vi "python_pattern_script_node.vi"(1 "Pattern Definition":T1={"Spot pitch (pixels)"=23.1, "Tilt Angle (deg)"=0.0, "Horizontal Offset (pixels)"=91.9, "Vertical Offset (pixels)"=14.1, "# Horizontal Spots"=8, "# Vertical Spots"=1, "Spot size (pixels)"=23.1, "Darken center spot"=FALSE, "Exact Phase Formula"=TRUE, "phase wrapping"=FALSE, "Set Focus (mm)"=32.0, "Add phase"=4.0, "phase_factor"=65.0, "Steering LW"=2.0, "Steering vmax"=0.0, "phase_overshoot"=TRUE, "Focal shift param"=0.0, "x0 focal shift"=0.0, "y0 focal shift"=0.0, "hv_steering"=TRUE, "fixed"=TRUE, "Pad"=0.0, "dark_all"=FALSE, "nospot"=FALSE, "Laser wavelength"=6.28e-07} {"Laser wavelength" min=0.0 max=500.0 format="%^#.3e"; "Pad" min=0.0 max=500.0 step=1.0 format="%#.0g"; "y0 focal shift" min=0.0 max=500.0 format="%#.3g"; "x0 focal shift" min=0.0 max=500.0 format="%#.3g"; "Focal shift param" min=0.0 max=500.0 format="%#.3g"; "Steering vmax" min=0.0 max=500.0 format="%#.3g"; "Steering LW" min=0.0 max=500.0 format="%#.3g"; "phase_factor" min=0.0 max=500.0 format="%#.3f"; "Add phase" min=0.0 max=500.0 format="%#.3f"; "Set Focus (mm)" min=0.0 max=500.0 format="%#.3g"; "Spot size (pixels)" min=1.0 format="%.2g"; "# Vertical Spots" min=1 step=1; "# Horizontal Spots" min=1 step=1; "Vertical Offset (pixels)" format="%.2f"; "Horizontal Offset (pixels)" format="%.2f"; "Tilt Angle (deg)" min=-90.0 max=90.0 format="%.2g"; "Spot pitch (pixels)" min=1.0 format="%.2g"}) -> (0 "Float Matrix":dbl[][](array[numeric]))   [LabVIEW 2011]
uses:
  Periodic Spot Pattern Parameters.ctl
  Periodic Spot Pattern Parameters2.ctl
panel:
  in  "center_spot (to be darkened)":u16=4
  in  "error in":errorcluster
  out "A string returned from the ScriptNode (debugging)":string="C:\\Data\\Antonio\\software\\LCOS\\LCOS"
  out "Xm":dbl[](array[numeric])=[21.72, 44.87, 68.2, 91.45, 114.72, 137.87, 160.97, 184.04]
  in  "Xm String (csv)":string="21.72,  44.87,  68.20,  91.45, 114.72, 137.87, 160.97, 184.04"
  out "Ym":dbl[](array[numeric])=[13.84, 13.78, 13.79, 13.83, 13.75, 13.79, 13.74, 13.68]
  in  "Ym String (csv)":string="13.84,  13.78,  13.79,  13.83,  13.75,  13.79,  13.74,  13.68"
  out "Intensity Graph":dbl[][](graph)
  out "error out":errorcluster
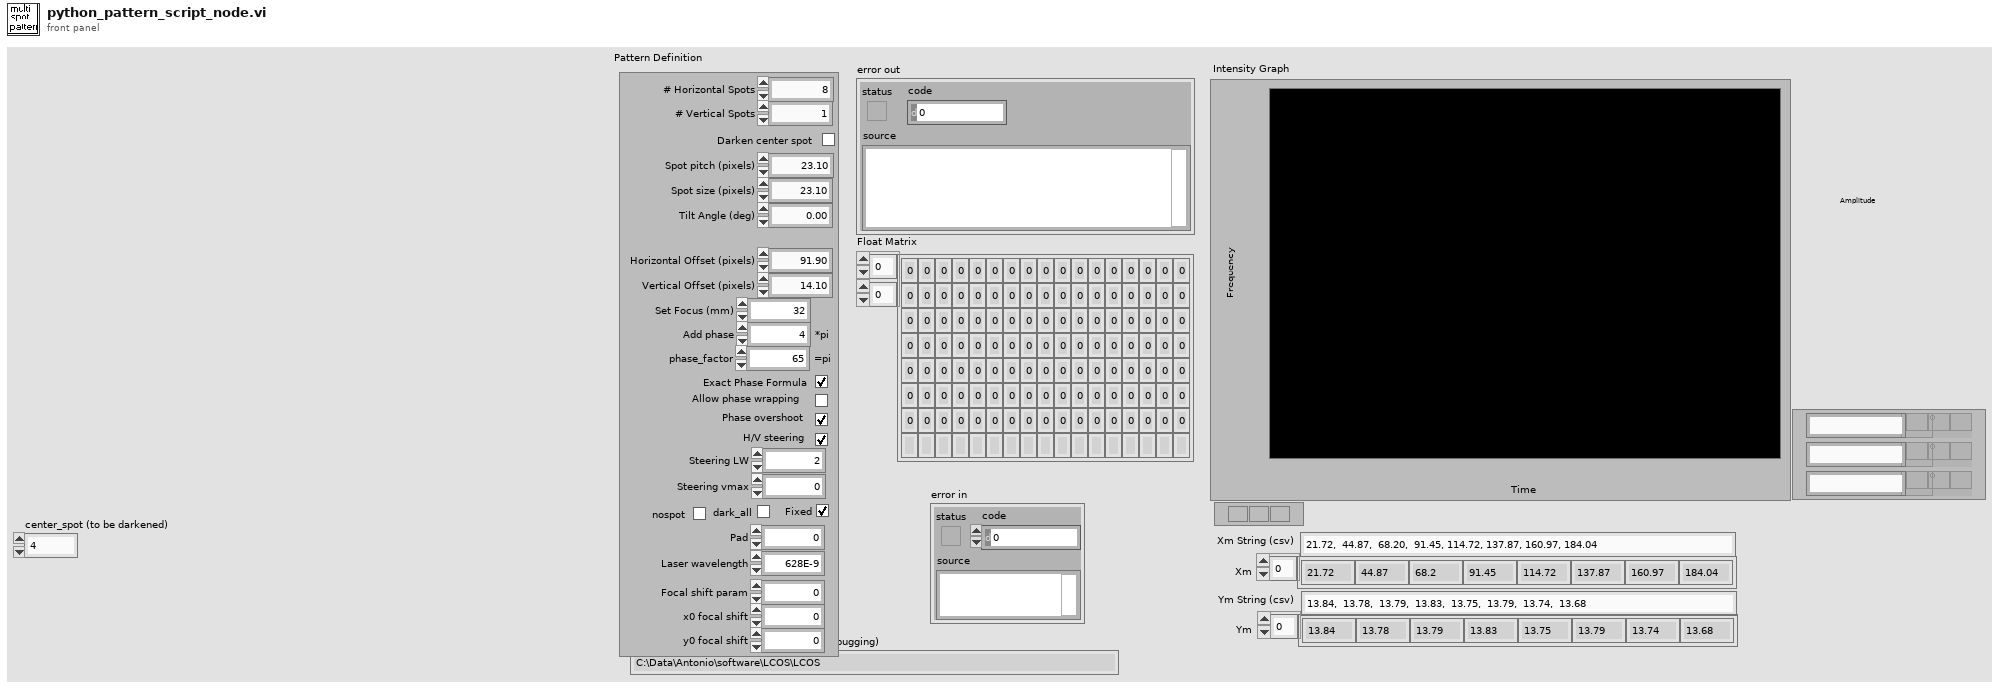
[diagram p1: front panel]
types:
  T1 = typedef "Periodic Spot Pattern Parameters.ctl" = cluster{"Spot pitch (pixels)":dbl, "Tilt Angle (deg)":dbl, "Horizontal Offset (pixels)":dbl, "Vertical Offset (pixels)":dbl, "# Horizontal Spots":u32, "# Vertical Spots":u32, "Spot size (pixels)":dbl, "Darken center spot":bool, "Exact Phase Formula":bool, "phase wrapping":bool, "Set Focus (mm)":T2, "Add phase":dbl, "phase_factor":dbl, "Steering LW":T2, "Steering vmax":T2, "phase_overshoot":bool, "Focal shift param":T2, "x0 focal shift":T2, "y0 focal shift":T2, "hv_steering":bool, "fixed":bool, "Pad":T2, "dark_all":bool, "nospot":bool, "Laser wavelength":dbl}
  T2 = typedef "Periodic Spot Pattern Parameters2.ctl" = dbl
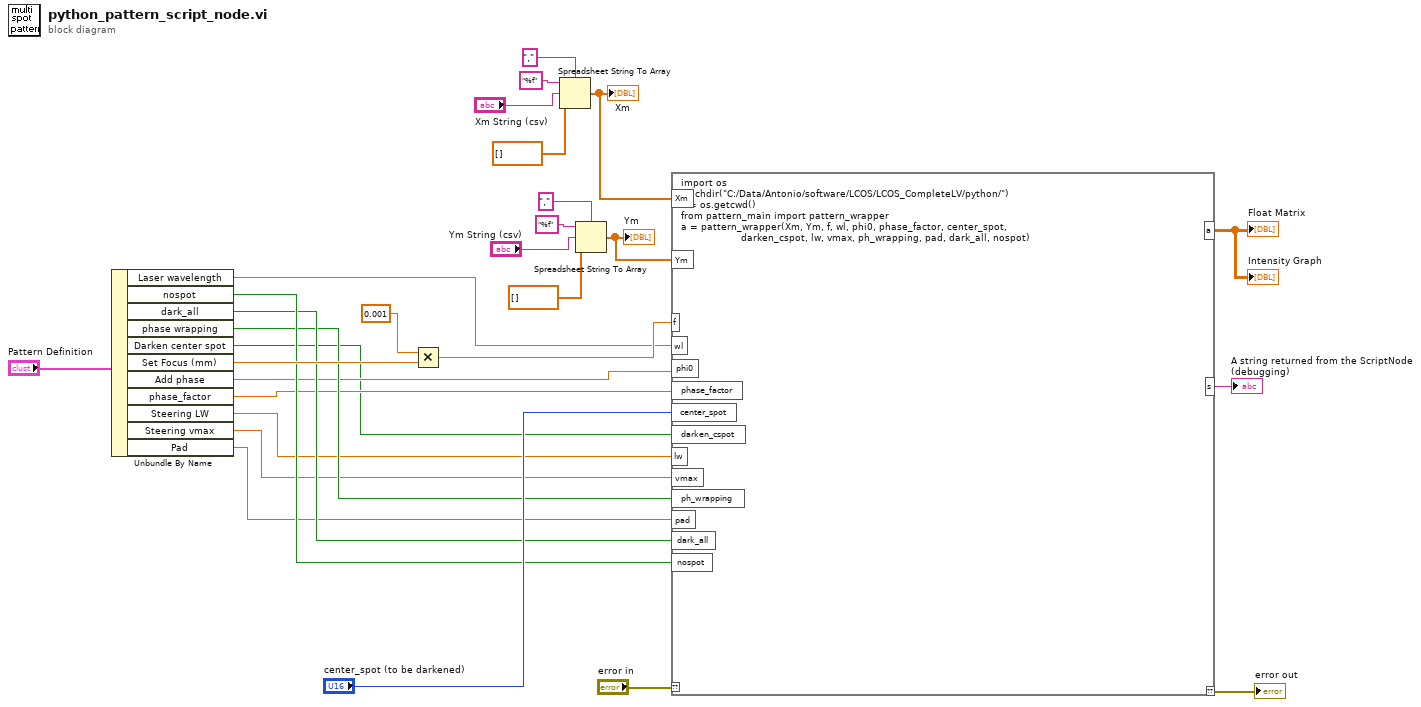
[diagram p0: block diagram]
diagram:
  n1 = Unbundle By Name("Pattern Definition") -> ("Laser wavelength"=w1:dbl, "nospot"=w10:bool, "dark_all"=w9:bool, "phase wrapping"=w8:bool, "Darken center spot"=w5:bool, "Set Focus (mm)"=w14:T2, "Add phase"=w7:dbl, "phase_factor"=w6:dbl, "Steering LW"=w4:T2, "Steering vmax"=w3:T2, "Pad"=w2:T2)
  n2 = Multiply(x=T2 0.001, y=w14) -> (x*y=w12:T2)
  n3 = Spreadsheet String To Array(delimiter (Tab)=",", format string="%f", spreadsheet string="Xm String (csv)", array type (2D Dbl)=dbl[] []) -> (array=w18:dbl[])
  "Xm" <- w18
  n4 = Spreadsheet String To Array(delimiter (Tab)=",", format string="%f", spreadsheet string="Ym String (csv)", array type (2D Dbl)=dbl[] []) -> (array=w23:dbl[])
  "Ym" <- w23
  n5 = script code="import os\nos.chdir(\"C:/Data/Antonio/software/LCOS/LCOS_CompleteLV/python/\")\ns = os.getcwd()\nfrom pattern_main import pattern_wrapper\na = pattern_wrapper(Xm, Ym, f, wl, phi0, phase_factor, center_spot, \n                    darken_cspot, lw, vmax, ph_wrapping, pad, dark_all, nospot)"("??"="error in", "f"=w12, "wl"=w1, "phi0"=w7, "phase_factor"=w6, "Xm"=w18, "Ym"=w23, "center_spot"="center_spot (to be darkened)", "darken_cspot"=w5, "lw"=w4, "vmax"=w3, "ph_wrapping"=w8, "pad"=w2, "dark_all"=w9, "nospot"=w10) -> ("??"=→"error out":errorcluster, "a"=→"Float Matrix" →"Intensity Graph":dbl[][], "s"=→"A string returned from the ScriptNode (debugging)":string)
